vi "Get Remaining Position.vi"(4 "error in (no error)":errorcluster, 6 "Axis In":i16, 7 "Controller Reference":refnum<k7>) -> (0 "error out":errorcluster, 1 "Position Remaining":sgl, 2 "Axis Out":i16, 3 "Controller Reference out":refnum<k7>)   [LabVIEW 2015]
doc: "Gets the input Axis Remaining Position. Remaining Position is the difference between the Current Position and the Target Position."
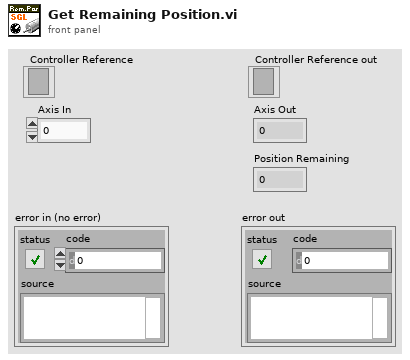
[diagram p1: front panel]
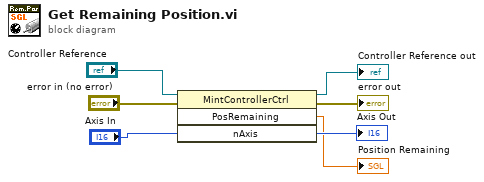
[diagram p0: block diagram]
diagram:
  n1 = invoke class="MintControllerCtrl" method="PosRemaining"(reference="Controller Reference", error in="error in (no error)", "nAxis"="Axis In") -> (reference out=→"Controller Reference out":refnum<k7>, error out=→"error out":errorcluster, "PosRemaining"=→"Position Remaining":sgl, "nAxis"=→"Axis Out":i16)  [unwired: 1 in]
